vi "RT Main.vi"() -> ()   [LabVIEW 2021]
doc: "This example generates two waveforms on the FPGA, transfers them to the CPU using DMA, and displays the waveforms."
uses:
  <vilib>/Platform/TimedLoop/XDataNode/timing_clust.ctl
  <vilib>/Platform/TimedLoop/XDataNode/nitl_modes.ctl
  <vilib>/Platform/TimedLoop/XDataNode/wakeup.ctl
  <vilib>/FPGAPlugInAG/myRIO-1900/niLvFpga_Open_myRIO-1900.vi
  <vilib>/rvi/interface/common/dynamic/niFpgaDynamicAddResources.vi
  <vilib>/rvi/interface/common/niFpgaWaitOnOcc.vi
  <vilib>/Utility/error.llb/Error Cluster From Error Code.vi
  <vilib>/rvi/errors/niLvFpgaAdjustHostInterfaceError.vi
  <vilib>/myRIO/Common/Instrument Driver Framework/Utilities/vis/FPGA Ref Manager.vi
  <vilib>/myRIO/Common/Instrument Driver Framework/Utilities/vis/Ref Counter.vi
  <vilib>/FPGAPlugInAG/Dynamic/niLvFpga_Run_Dynamic.vi
  <vilib>/rvi/Analysis/host/Private/Sample Rate To Loop Time (ticks).vi
  <vilib>/rvi/Analysis/host/Notch/config/NotchScaledCoefficients.vi
  <vilib>/FPGAPlugInAG/Dynamic/niLvFpga_Abort_Dynamic.vi
  <vilib>/FPGAPlugInAG/Dynamic/niLvFpga_Close_Dynamic.vi
  <vilib>/rvi/interface/nirviOpenFPGA/nirviOpenFPGA.xnode
  FPGA Bitfiles/SignalGenerator.lvbitx
  <vilib>/rvi/interface/nirviMethod/nirviMethod.xnode
  <vilib>/rvi/interface/nirviReadWriteControl/nirviReadWriteControl.xnode
  <vilib>/Platform/TimedLoop/XDataNode/XDataNode.xnode
  <vilib>/rvi/Analysis/host/Notch/XNode/NotchCoefficients.xnode
  <vilib>/rvi/interface/nirviCloseFPGA/nirviCloseFPGA.xnode
  <vilib>/rvi/errors/niLvFpgaMergeErrorWithErrorCode.vi
  <vilib>/rvi/Analysis/host/Public/NI_FpgaMspHost.lvlib
  <vilib>/rvi/interface/Simulation/niFpgaSimulationCallBeginRW.vi
  <vilib>/myRIO/Instrument Drivers/Utilities/Utilities.lvlib
  <vilib>/Platform/TimedLoop/XDataNode/XDNodeRunTimeDep.lvlib
  NiFpgaLv.dll
  <vilib>/FPGAPlugInAG/Dynamic/niLvFpga_ConfigureFifo_Dynamic.vi
  <vilib>/FPGAPlugInAG/Dynamic/niLvFpga_StartFifo_Dynamic.vi
  <vilib>/FPGAPlugInAG/Dynamic/niLvFpga_ReadFifo_Dynamic.vi
panel:
  out "End?":bool
  out "error out":errorcluster
  in  "Stop":bool
  in  "Tab Control":enum32{"SineWave", "Filtered Sine Wave (A/AO1)"}(tab)
  out "Sine Wave":waveform(ext)(graph)
  in  "Sine Wave Parameters":T1={"Frequency (Hz)"=1000.0, "Phase offset (deg)"=0.0, "Vpeak (V)"=5.0, "Offset (V)"=0.0} {"Phase offset (deg)" format="%#_6p"; "Frequency (Hz)" format="%#_6p"}
  out "Filtered Sine Wave":waveform(ext)(graph)
  in  "Filter Coefficient":T2={"Notch Frequency (Hz)"=1000.0, "Q factor"=5.0} {"Q factor" format="%#_6f"; "Notch Frequency (Hz)" format="%#_6p"}
  # "Overview: This example generates two waveforms on the FPGA, transfers them to the CPU using DMA, and displays the waveforms. This example ships with an FPGA bitfile. If you modify the FPGA code you must recompile the FPGA code.\nRequirements: \n1. myRIO-1900\n2. LabVIEW FPGA Module\n3. Xilinx Compilation Tools. \nInstructions:\n1. Check the myRIO target IP Address in the project and make sure the target IP Address is correct. \n2. Run the VI. \n3. Change the waveform parameters on the tabs. This VI reads the waveforms simultaneously. \n4. The FPGA outputs the waveforms on two channels: connectors A/AO0 and A/AO1.\n5. The Open FPGA VI Reference in this example points directly to the FPGA bitfile. If you make changes to the FPGA code, LabVIEW may not notify you that a rebuild of the FPGA code is necessary. You can change this behavior by modifying the Open FPGA VI Reference to point to the FPGA VI or the FPGA Build Specification. Caution: You may then need to rebuild the FPGA code."
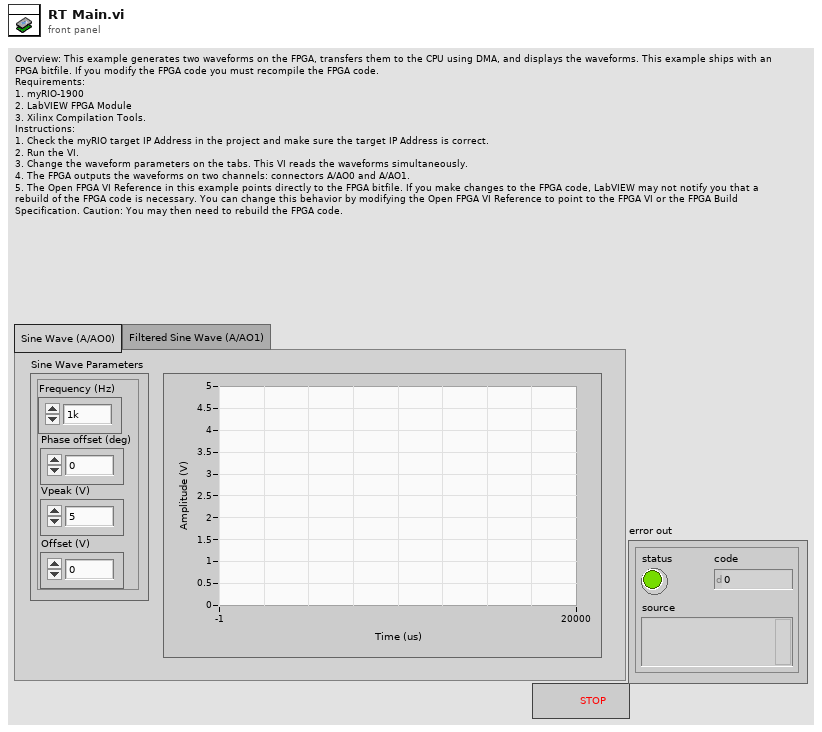
[diagram p1: front panel]
types:
  T1 = cluster{"Frequency (Hz)":dbl, "Phase offset (deg)":dbl, "Vpeak (V)":dbl, "Offset (V)":dbl}
  T2 = cluster{"Notch Frequency (Hz)":dbl, "Q factor":dbl}
  T3 = cluster{"read mode":enum16{"polling", "blocking"}, "write mode":enum16{"polling", "blocking"}}
  T4 = cluster{"Frequency (periods/tick)":dbl, "Phase offset (periods)":dbl, "Scale factor":dbl, "Amplitude offset":dbl}
  T5 = typedef "XDNodeRunTimeDep.lvlib/timing_clust.ctl" = cluster{"Expected End [f-1]":u64, "Actual End [f-1]":u64, "Finished Late? [f-1]":bool, "Expected End [i-1]":u64, "Actual End [i-1]":u64, "Finished Late? [i-1]":bool, "Expected Start [i]":u64, "Actual Start [i]":u64, "Expected Start [f]":u64, "Actual Start [f]":u64, "Source Name":string, "Structure Name":string, "Period":i64, "Deadline":i64, "Offset":i64, "Start":i64, "Priority":i32, "Timeout":i32, "Mode":T6, "Wakeup Reason":T7, "Error":errorcluster, "Source Type":string, "Secondary Source Type":string, "Global End Time":u64, "Global Start Time":u64, "Frame Duration":u64, "Iteration Duration":u64, "Assigned CPU":i32, "I/O Scan Engine Mode":u32}
  T6 = typedef "XDNodeRunTimeDep.lvlib/nitl_modes.ctl" = enum32{"No Change", "Process missed periods, maintain original phase", "Discard missed periods, maintain original phase", "Process missed periods, ignore original phase", "Discard missed periods, ignore original phase"}
  T7 = typedef "XDNodeRunTimeDep.lvlib/wakeup.ctl" = enum32{"Normal", "Aborted", "Asynchronous wakeup", "Timing source error", "Timed loop error", "Timeout"}
  T8 = cluster{"Notch Frequency (Hz)":bool, "Q factor":bool}
  T9 = cluster{"Frequency (periods/tick)":fxp<+,32,0>, "Phase offset (periods)":fxp<+,32,0>, "Scale factor":fxp<+,12,1>, "Amplitude offset":fxp<+/-,16,12>}
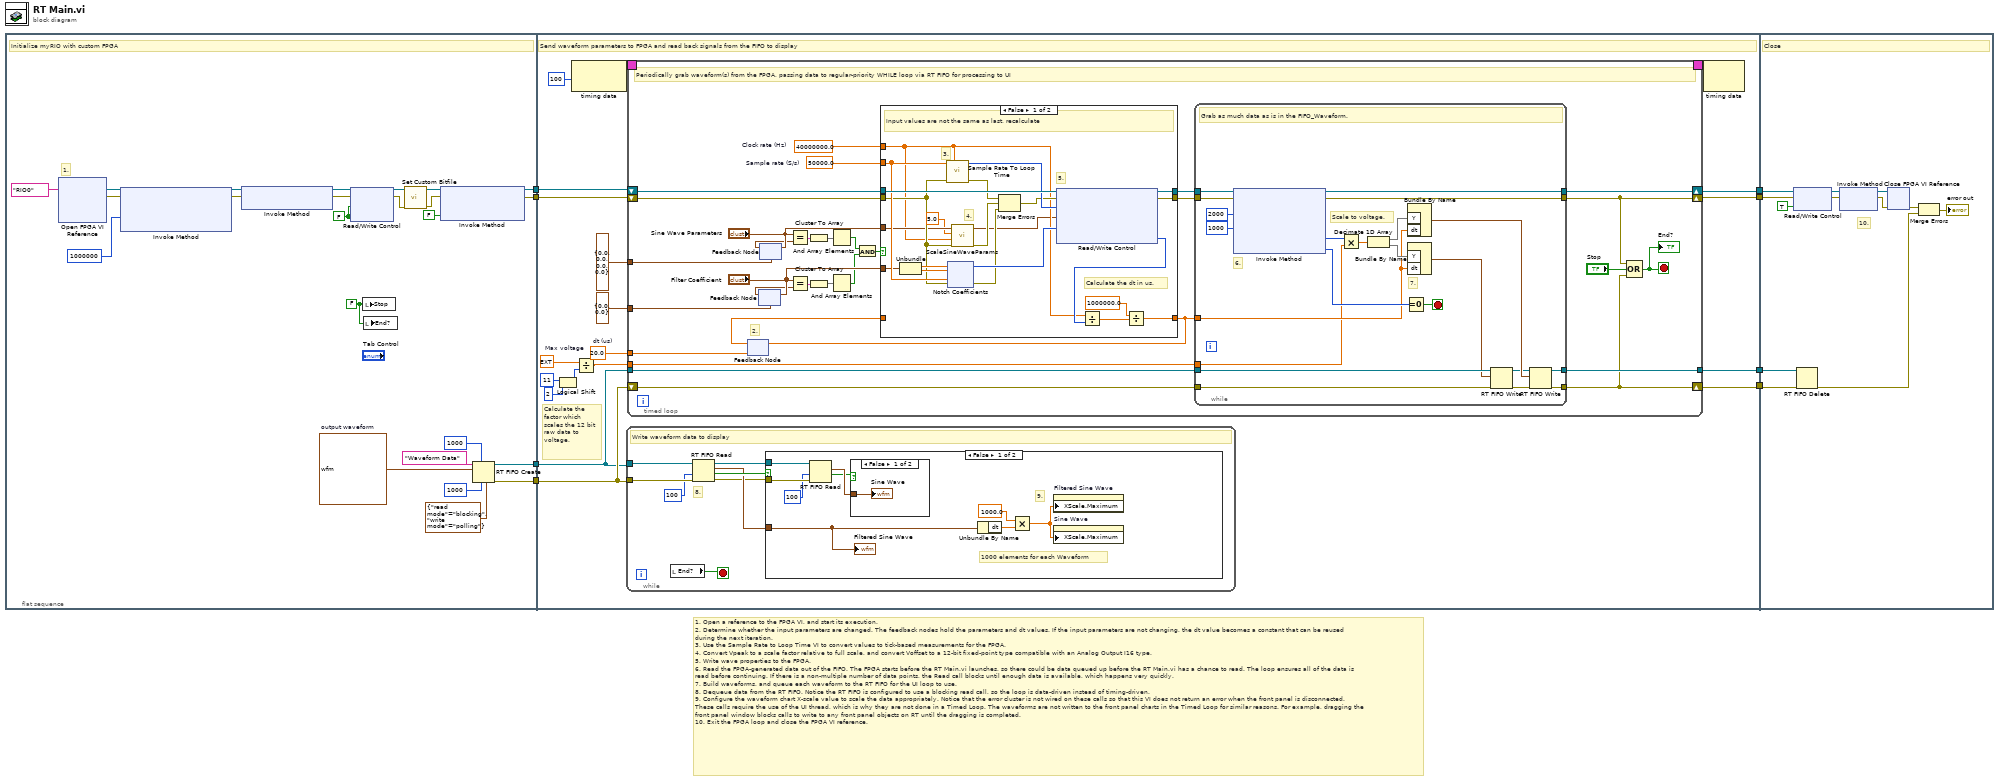
[diagram p0: block diagram]
diagram:
  # "1. Open a reference to the FPGA VI, and start its execution.\n2. Determine whether the input parameters are changed. The feedback nodes hold the parameters and dt values. If the input parameters are not changing, the dt value becomes a constant that can be reused during the next iteration.\n3. Use the Sample Rate to Loop Time VI to convert values to tick-based measurements for the FPGA.\n4. Convert Vpeak to a scale factor relative to full scale, and convert Voffset to a 12-bit fixed-point type compatible with an Analog Output I16 type.\n5. Write wave properties to the FPGA. \n6. Read the FPGA-generated data out of the FIFO. The FPGA starts before the RT Main.vi launches, so there could be data queued up before the RT Main.vi has a chance to read. The loop ensures all of the data is read before continuing. If there is a non-multiple number of data points, the Read call blocks until enough data is available, which happens very quickly.\n7. Build waveforms, and queue each waveform to the RT FIFO for the UI loop to use.\n8. Dequeue data from the RT FIFO. Notice the RT FIFO is configured to use a blocking read call, so the loop is data-driven instead of timing-driven.\n9. Configure the waveform chart X-scale value to scale the data appropriately. Notice that the error cluster is not wired on these calls so that this VI does not return an error when the front panel is disconnected. These calls require the use of the UI thread, which is why they are not done in a Timed Loop. The waveforms are not written to the front panel charts in the Timed Loop for similar reasons. For example, dragging the front panel window blocks calls to write to any front panel objects on RT until the dragging is completed.\n10. Exit the FPGA loop and close the FPGA VI reference."
  n1 = flat-sequence {
    tunnel: [w19] -> w8
    tunnel: [w18] -> w7
    tunnel: [w14] -> w4
    tunnel: [w13] -> w3
    tunnel: w8 -> [w51]
    tunnel: w7 -> [w50]
    tunnel: [w49] -> w6
    tunnel: [w40] -> w5
    tunnel: w4 -> [w45]
    tunnel: w3 -> [w46]
    tunnel: [w41] -> w2
    tunnel: [w39] -> w1
    tunnel: w6 -> [w171]
    tunnel: w5 -> [w164]
    tunnel: w2 -> [w166]
    tunnel: w1 -> [w165]
    frame #0 {
      w10 = waveform(ext) {"t0"=timestamp(0 s since 1904-01-01), "dt"=1.0, "Y"=[]}  # output waveform
      w12 = FALSE ("Reset")
      w26 = FALSE ("Stop")
      # "1."
      # "Initialize myRIO with custom FPGA"
      n2 = xnode "Open FPGA VI Reference"("resource name"=tag "RIO0") -> ("FPGA VI Reference Out"=w24:refnum<k20>, "error out"=w23:errorcluster)  [unwired: 1 in]
      n3 = xnode "Invoke Method"("FPGA VI Reference In"=w24, "error in"=w23, "Requested Depth"=u32 1000000) -> ("FPGA VI Reference Out"=w30:refnum<k20>, "error out"=w29:errorcluster)  [unwired: 1 out]
      n4 = xnode "Invoke Method"("FPGA VI Reference In"=w30, "error in"=w29) -> ("FPGA VI Reference Out"=w28:refnum<k20>, "error out"=w27:errorcluster)
      n5 = xnode "Read/Write Control"("FPGA VI Reference In"=w28, "error in"=w27, "Stop"=w26, "Initialize"=w26) -> ("FPGA VI Reference Out"=w25:refnum<k20>, "error out"=w22:errorcluster)
      n6 = local write "Stop"(w12) -> ()
      n7 = local write "End?"(w12) -> ()
      n8 = call <vilib>:"Set Custom Bitfile.vi"("error in (no error)"=w22, "Custom FPGA Reference In"=w25) -> ("error out"=w20:errorcluster, "Custom FPGA Reference Out"=w21:refnum<k20>)  [unwired: 8 in]
      n9 = xnode "Invoke Method"("FPGA VI Reference In"=w21, "error in"=w20, "Wait Until Done (F)"=FALSE) -> ("FPGA VI Reference Out"=w19:refnum<k20>, "error out"=w18:errorcluster)
      n10 = RT FIFO Create(0:"Waveform Data" ("name (unnamed)"), 1:w10, 4:u32 1000 ("size (10)"), 5:u32 1000 ("datapoints in waveform (1)"), 7:T3 {"read mode"=enum."blocking", "write mode"=enum."polling"} ("r/w modes (polling,polling)")) -> (8:w14:refnum<k33>, 11:w13:errorcluster)  [unwired: 3 in, 1 out]
    }
    frame #1 {
      w35 = ext 5.0  # Max voltage
      w38 = 20.0  # dt (us)
      # "Calculate the factor which scales the 12 bit raw data to voltage."
      # "Send waveform parameters to FPGA and read back signals from the FIFO to display"
      n11 = Logical Shift(y=i16 11, x=i16 2) -> (x << y=w34:i16)
      n12 = node-c288(i64 100 ("Period")) -> (w48:T5)
      n13 = Divide(x=w35, y=w34) -> (x/y=w33:ext)
      n14 = while {
        tunnel: w46 -> [w57]
        tunnel: w45 -> [w58]
        stop <- w59 stop-if-true
        # "8."
        # "Write waveform data to display"
        n15 = local read "End?"() -> (w59:bool)
        n16 = RT FIFO Read(0:w58, 2:100 ("timeout in ms (0)"), 3:w57) -> (8:w53:refnum<k33>, 9:w55:waveform(ext), 10:w56:bool, 11:w52:errorcluster)  [unwired: 1 in, 1 out]
        n17 = case shown="False" w56 {
          tunnel: w55 -> [w63 _]
          tunnel: w53 -> [w67 _]
          tunnel: w52 -> [w68 _]
          frame False {
            # "9."
            # "1000 elements for each Waveform"
            n18 = RT FIFO Read(0:w67, 2:100 ("timeout in ms (0)"), 3:w68) -> (9:w66:waveform(ext), 10:w60:bool)  [unwired: 1 in, 3 out]
            n19 = case shown="False" w60 {
              tunnel: w66 -> [w69 _]
              frame False {
                "Sine Wave" <- w69
              }
              frame True {
              }
            }
            n20 = Unbundle By Name(w63) -> ("dt"=w62:dbl)
            n21 = Multiply(x=1000.0, y=w62) -> (x*y=w64:dbl)
            n22 = property on="Filtered Sine Wave" class="WFGraph (strict)"("XScale.Maximum"=w64) -> ()  [unwired: 2 in, 2 out]
            n23 = property on="Sine Wave" class="WFGraph (strict)"("XScale.Maximum"=w64) -> ()  [unwired: 2 in, 2 out]
            "Filtered Sine Wave" <- w63
          }
          frame True {
          }
        }
      }
      n24 = timed-loop {
        shift-right: [w87] -> w40
        shift-left: w50 -> [w97]
        shift-right: [w100] -> w49
        shift-left: w51 -> [w99]
        timing: w48 -> [_]
        timing-out: [_] -> w47
        tunnel: w45 -> [w92]
        tunnel: [w91] -> w41
        shift-right: [w88] -> w39
        shift-left: w46 -> [w93]
        tunnel: T4 {"Frequency (periods/tick)"=0.0, "Phase offset (periods)"=0.0, "Scale factor"=0.0, "Amplitude offset"=0.0} ("Sinewave Props") -> [w84]
        tunnel: T2 {"Notch Frequency (Hz)"=0.0, "Q factor"=0.0} ("Filter Coefficient") -> [w83]
        tunnel: w38 -> [w73]
        tunnel: w33 -> [w70]
        stop <- w89 stop-if-true
        w98 = 50000.0  # Sample rate (S/s)
        w94 = 40000000.0  # Clock rate (Hz)
        # "2."
        # "Periodically grab waveform(s) from the FPGA, passing data to regular-priority WHILE loop via RT FIFO for processing to UI"
        n25 = feedback #1(w73) -> (w71:dbl)
        n26 = feedback #2(w83) -> (w74:T2)
        n27 = feedback-in #2("Filter Coefficient") -> ()
        n28 = feedback #3(w84) -> (w76:T4)
        n29 = feedback-in #3("Sine Wave Parameters") -> ()
        n30 = Equal?(x="Filter Coefficient", y=w74) -> (x = y?=w81:T8)
        n31 = Equal?(x="Sine Wave Parameters", y=w76) -> (x = y?=w80:cluster{bool, bool, bool, bool})
        n32 = Cluster To Array(cluster=w80) -> (array=w79:bool[])
        n33 = Cluster To Array(cluster=w81) -> (array=w78:bool[])
        n34 = And Array Elements(Boolean array=w79) -> (logical AND=w77:bool)
        n35 = And Array Elements(Boolean array=w78) -> (logical AND=w75:bool)
        n36 = And(x=w77, y=w75) -> (x .and. y?=w82:bool)
        n37 = case shown="False" w82 {
          tunnel: w99 -> [w122 w131]
          tunnel: w98 -> [w119 _]
          tunnel: "Filter Coefficient" -> [w101 _]
          tunnel: w97 -> [w112 w130]
          tunnel: "Sine Wave Parameters" -> [w111 _]
          tunnel: [w109 w131] -> w96
          tunnel: [w108 w130] -> w95
          tunnel: w94 -> [w104 _]
          tunnel: [w103 w132] -> w72
          tunnel: w71 -> [_ w132]
          frame False {
            # "3."
            # "Calculate the dt in us."
            # "5."
            # "4."
            # "Input values are not the same as last, recalculate"
            n38 = Unbundle(w101) -> ("Notch Frequency (Hz)"=w115:dbl, "Q factor"=w114:dbl)
            n39 = call-poly <vilib>:"Sample Rate To Loop Time.vi"("sample rate (S/s)"=w119, "FPGA clock rate (Hz)"=w104, "error in (no error)"=w112) -> ("count (ticks/S)"=w121:u32, "error out"=w113:errorcluster)  [unwired: 10 in, 1 out]
            n40 = xnode "Notch Coefficients"("notch frequency (Hz)"=w115, "Q factor"=w114, "sample rate (S/s)"=w119, "error in (no error)"=w112) -> ("scaled coefficients"=w120:i32[], "error out"=w117:errorcluster)
            n41 = call "ScaleSineWaveParams.vi"("error in (no error)"=w112, "FPGA Clock Rate"=w104, "max voltage for target"=5.0, "Sine wave"=w111) -> ("error out"=w118:errorcluster, "Sinewave Props"=w102:T9)  [unwired: 6 in]
            n42 = Merge Errors(w113, w118, w117) -> (w116:errorcluster)
            n43 = xnode "Read/Write Control"("FPGA VI Reference In"=w122, "error in"=w116, "Desired loop rate (ticks)"=w121, "Sine wave properties"=w102, "Filter scaled coefficients"=w120) -> ("FPGA VI Reference Out"=w109:refnum<k20>, "error out"=w108:errorcluster, "Actual loop rate"=w107:u32)
            n44 = Divide(x=w104, y=w107) -> (x/y=w105:dbl)
            n45 = Divide(x=1000000.0, y=w105) -> (x/y=w103:dbl)
          }
          frame True {
            # "Input values did not change, use previous values"
          }
        }
        n46 = feedback-in #1(w72) -> ()
        n47 = while {
          tunnel: [w154] -> w100
          tunnel: w96 -> [w151]
          tunnel: w95 -> [w150]
          tunnel: w93 -> [w149]
          tunnel: w92 -> [w148]
          tunnel: [w136] -> w91
          tunnel: w72 -> [w142]
          tunnel: [w138] -> w88
          tunnel: [w147] -> w87
          tunnel: w70 -> [w134]
          stop <- w146 stop-if-true
          # "Scale to voltage."
          # "7."
          # "6."
          # "Grab as much data as is in the FIFO_Waveform."
          n48 = xnode "Invoke Method"("FPGA VI Reference In"=w151, "error in"=w150, "Number of Elements"=u32 2000, "Timeout (ms)"=1000) -> ("FPGA VI Reference Out"=w154:refnum<k20>, "error out"=w147:errorcluster, "Data"=w135:u16[], "Elements Remaining"=w145:u32)
          n49 = Multiply(x=w135, y=w134) -> (x*y=w133:ext[])
          n50 = Decimate 1D Array(w133) -> (w144:ext[], w143:ext[])
          n51 = Equal To 0?(x=w145) -> (x = 0?=w146:bool)
          n52 = Bundle By Name("Y"=w144, "dt"=w142) -> (w140:waveform(ext))  [unwired: 1 in]
          n53 = Bundle By Name("Y"=w143, "dt"=w142) -> (w141:waveform(ext))  [unwired: 1 in]
          n54 = RT FIFO Write(0:w148, 1:w141, 3:w149) -> (8:w137:refnum<k33>, 11:w139:errorcluster)  [unwired: 2 in, 2 out]
          n55 = RT FIFO Write(0:w137, 1:w140, 3:w139) -> (8:w136:refnum<k33>, 11:w138:errorcluster)  [unwired: 2 in, 2 out]
        }
        n56 = Compound Arithmetic op=OR(w87, "Stop", w88) -> (w89:bool)
        "End?" <- w89
      }
      n57 = node-c288(w47) -> ()  [unwired: 1 out]
    }
    frame #2 {
      # "10."
      # "Close"
      n58 = xnode "Read/Write Control"("FPGA VI Reference In"=w171, "error in"=w164, "Stop"=TRUE) -> ("FPGA VI Reference Out"=w170:refnum<k20>, "error out"=w169:errorcluster)
      n59 = RT FIFO Delete(0:w166, 3:w165) -> (11:w162:errorcluster)  [unwired: 1 in]
      n60 = xnode "Invoke Method"("FPGA VI Reference In"=w170, "error in"=w169) -> ("FPGA VI Reference Out"=w168:refnum<k20>, "error out"=w167:errorcluster)
      n61 = xnode "Close FPGA VI Reference"("FPGA VI Reference In"=w168, "error in"=w167) -> ("error out"=w163:errorcluster)
      n62 = Merge Errors(w163, w162) -> (→"error out":errorcluster)
    }
  }
